vi "Create DVR_Occurrence.vi"(11 "error in (no error)":errorcluster) -> (4 "Without data DVR reference":refnum<data-value>, 15 "error out":errorcluster)   [LabVIEW 2020, in "Data Communication Transmitter.lvlib" / "Without Data.lvclass"]
uses:
  Classes/Children/Intra-Application/Children/Without data/Without Data.lvclass
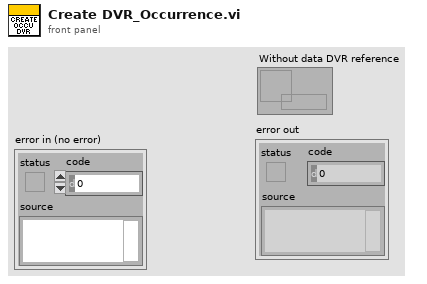
[diagram p1: front panel]
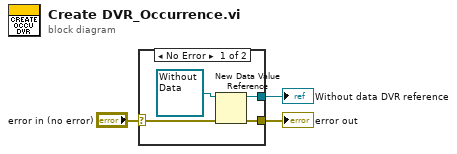
[diagram p0: block diagram]
diagram:
  n1 = case shown="No Error" "error in (no error)" {
    selector: "error in (no error)" -> [w7 w8]
    tunnel: [w6 w8] -> w2
    tunnel: [w5 _] -> w1
    frame No Error {
      n2 = New Data Value Reference(data value=refnum<class "Without Data.lvclass"> refnum ("Data Communication.lvlib:Without Data.lvclass"), error in=w7) -> (data value reference=w5:refnum<data-value>, error out=w6:errorcluster)
    }
    frame Error {
    }
  }
  "error out" <- w2
  "Without data DVR reference" <- w1
